vi "test_suite_log.vi"() -> ()   [LabVIEW 2010]
uses:
  protocol_Generic/Protocol_Generic.lvclass
  protocol_A/Protocol_a.lvclass
  protocol_B/Protocol_B.lvclass
  protocol_MoveToSetpoint/Protocol_MoveToSetpoint.lvclass
panel:
  out "error out":errorcluster
  in  "error in (no error)":errorcluster
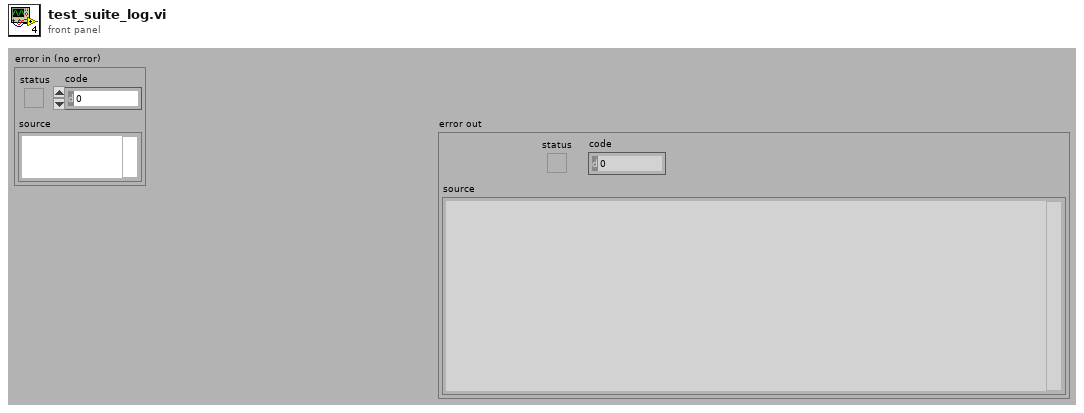
[diagram p1: front panel]
types:
  T1 = cluster{"Protocol_Generic.lvclass":refnum<class "Protocol_Generic.lvclass">}[]
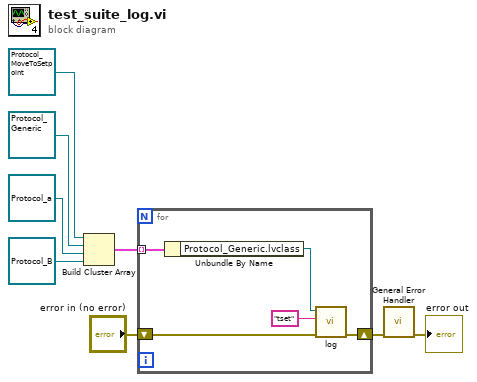
[diagram p0: block diagram]
diagram:
  n1 = Build Cluster Array(refnum<class "Protocol_MoveToSetpoint.lvclass"> refnum ("Protocol_MoveToSetpoint.lvclass"), refnum<class "Protocol_Generic.lvclass"> refnum ("Protocol_Generic.lvclass"), refnum<class "Protocol_a.lvclass"> refnum ("Protocol_A.lvclass"), refnum<class "Protocol_B.lvclass"> refnum ("Protocol_B.lvclass")) -> (w7:T1)
  n2 = for {
    tunnel: w7 -> [w13] mode=indexing
    shift-right: [w10] -> w1
    shift-left: "error in (no error)" -> [w11]
    n3 = Unbundle By Name(w13) -> ("Protocol_Generic.lvclass"=w12:refnum<class "Protocol_Generic.lvclass">)
    n4 = call-dynamic "log.vi"("error in (no error)"=w11, "logLineIn"="tset", "Protocol_Generic in"=w12) -> ("error out"=w10:errorcluster)  [unwired: 7 in, 1 out]
  }
  n5 = call <vilib>:"General Error Handler.vi"("error in (no error)"=w1) -> ("error out"=→"error out":errorcluster)  [unwired: 10 in, 4 out]
